vi "Untitled 3 (SubVI).vi"(11 "Serial Init":T1={"Puerto Serial"="", "baud rate (9600)"=9600, "data bits (8)"=8, "parity (0:none)"=enum."None", "error in (no error)"={"status"=FALSE, "code"=0, "source"=""}, "stop bits (10: 1 bit)"=10, "flow control (0:none)"=0} {"flow control (0:none)" items=["None", "XON/XOFF", "RTS/CTS", "XON/XOFF & RTS/CTS", "DTR/DSR", "XON/XOFF & DTR/DSR"]; "stop bits (10: 1 bit)" items=["1.0"=10, "1.5"=15, "2.0"=20]; "data bits (8)" min=5 max=8 step=1}) -> (0 "error out":errorcluster, 3 "VISA Refnum out":refnum<visa-resource-name>)   [LabVIEW 2020]
uses:
  <vilib>/Instr/_visa.llb/VISA Configure Serial Port (Instr).vi
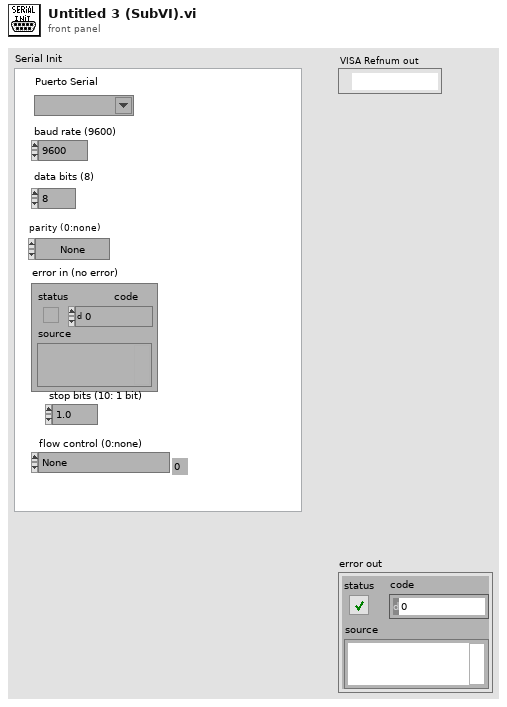
[diagram p1: front panel]
types:
  T1 = cluster{"Puerto Serial":refnum<visa-resource-name>, "baud rate (9600)":u32, "data bits (8)":u16, "parity (0:none)":enum16{"None", "Odd", "Even", "Mark", "Space"}, "error in (no error)":errorcluster, "stop bits (10: 1 bit)":u16, "flow control (0:none)":u16}
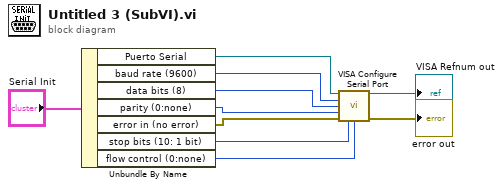
[diagram p0: block diagram]
diagram:
  n1 = Unbundle By Name("Serial Init") -> ("Puerto Serial"=w2:refnum<visa-resource-name>, "baud rate (9600)"=w3:u32, "data bits (8)"=w4:u16, "parity (0:none)"=w5:enum16{"None", "Odd", "Even", "Mark", "Space"}, "error in (no error)"=w6:errorcluster, "stop bits (10: 1 bit)"=w7:u16, "flow control (0:none)"=w8:u16)
  n2 = call-poly "VISA Configure Serial Port"("VISA resource name"=w2, "baud rate (9600)"=w3, "data bits (8)"=w4, "parity (0:none)"=w5, "error in (no error)"=w6, "stop bits (10: 1 bit)"=w7, "flow control (0:none)"=w8) -> ("VISA resource name out"=→"VISA Refnum out":refnum<visa-resource-name>, "error out"=→"error out":errorcluster)  [unwired: 7 in]
